vi "Tester_Sensor_data_to_value.vi"() -> ()   [LabVIEW 2013]
panel:
  out "Slide 2":u16(slide) scale=0.0..65536.0
  out "Slide":u8(slide) scale=0.0..255.0
  out "ok?":bool
  # "FULL COVERAGE TEST FOR DATA COVERTER OLD AND NEW VERSION"
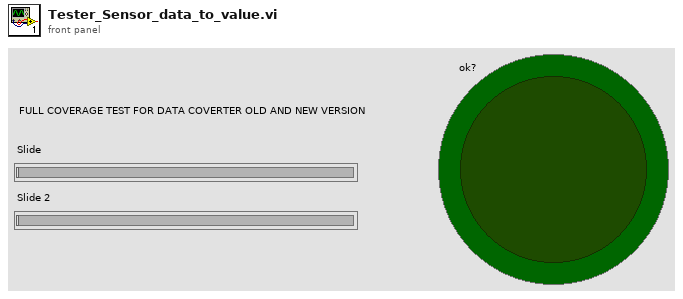
[diagram p1: front panel]
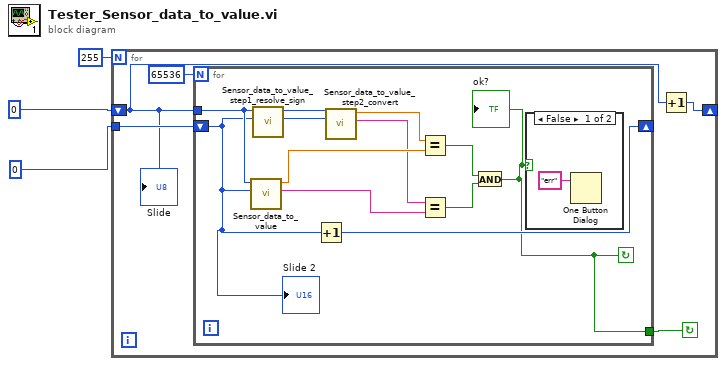
[diagram p0: block diagram]
diagram:
  n1 = for {
    N: 255 -> [_]
    tunnel: u16 0 ("Sensor data") -> [w8]
    shift-right: [w7] -> _
    shift-left: u8 0 ("Sensor type") -> [w4]
    stop <- w5 continue-if-true
    n2 = for {
      N: 65536 -> [_]
      tunnel: w4 -> [w12]
      shift-right: [w11] -> _
      shift-left: w8 -> [w9]
      tunnel: [w10] -> w5
      stop <- w10 continue-if-true
      n3 = call "Sensor_data_to_value.vi"("Sensor data"=w9, "Sensor type"=w12) -> ("Signal legend"=w15:string, "Value ouptut"=w17:dbl)  [unwired: 7 in, 1 out]
      n4 = call "Sensor_data_to_value_step1_resolve_sign.vi"("Sensor data"=w9, "Sensor type"=w12) -> ("Sensor data resolved sign"=w19:i32, "Sensor type out"=w20:u8)  [unwired: 8 in]
      n5 = Increment(x=w9) -> (x+1=w11:u16)
      n6 = call "Sensor_data_to_value_step2_convert.vi"("Sensor data resolved sign"=w19, "Sensor type"=w20) -> ("Signal legend"=w16:string, "Value ouptut"=w18:dbl)  [unwired: 8 in]
      n7 = Equal?(x=w18, y=w17) -> (x = y?=w14:bool)
      n8 = Equal?(x=w16, y=w15) -> (x = y?=w13:bool)
      n9 = And(x=w14, y=w13) -> (x .and. y?=w10:bool)
      "ok?" <- w10
      n10 = case shown="False" w10 {
        frame False {
          n11 = One Button Dialog(message="err") -> ()  [unwired: 1 in, 1 out]
        }
        frame True {
        }
      }
      "Slide 2" <- w9
    }
    n12 = Increment(x=w4) -> (x+1=w7:u8)
    "Slide" <- w4
  }
